vi "Cleanup Session.vi"(8 "error in":errorcluster, 11 "Plugin in":refnum<class "DateTimeChannel.lvclass">) -> (0 "error out":errorcluster, 3 "Plugin out":refnum<class "DateTimeChannel.lvclass">)   [LabVIEW 2023, in "DateTimeChannel.lvlib" / "DateTimeChannel.lvclass"]
uses:
  DateTimeChannel.lvclass
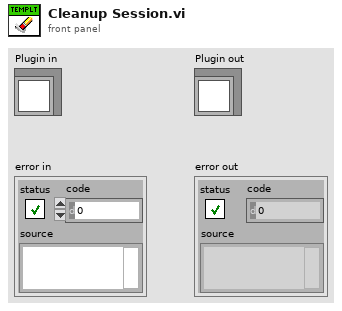
[diagram p1: front panel]
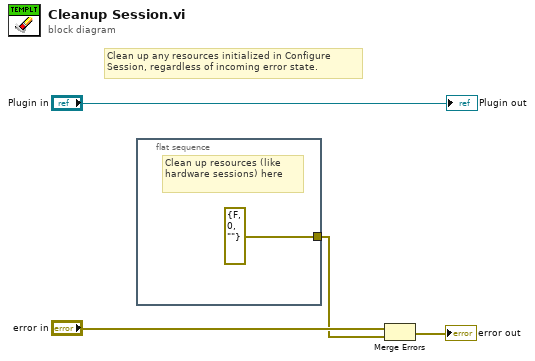
[diagram p0: block diagram]
diagram:
  # "Clean up any resources initialized in Configure Session, regardless of incoming error state."
  n1 = flat-sequence {
    tunnel: [errorcluster {"status"=FALSE, "code"=0, "source"=""} ("error in")] -> w1
    frame #0 {
      # "Clean up resources (like hardware sessions) here"
    }
  }
  n2 = Merge Errors("error in", w1) -> (→"error out":errorcluster)
  "Plugin out" <- "Plugin in"
